vi "Find Object Layout Index by UID.vi"(8 "error in (no error)":errorcluster, 9 "unique name":i32, 10 "object ID list in":variant, 11 "object layouts in":refnum<class "Object Layout.lvclass">[](array[class])) -> (0 "error out":errorcluster, 1 "found?":bool, 2 "object ID list out":variant, 3 "object layouts out":refnum<class "Object Layout.lvclass">[](array[class]), 5 "object layout index":i32)   [LabVIEW 2010, in "NI_SE_Front Panel Layout.lvlib"]
uses:
  NI_SE_Front Panel Layout.lvlib
  Object Layout Classes/Object Layout/Object Layout.lvclass
  Object Layout Classes/Object Layout/Object Layout.lvclass/Object Layout.ctl
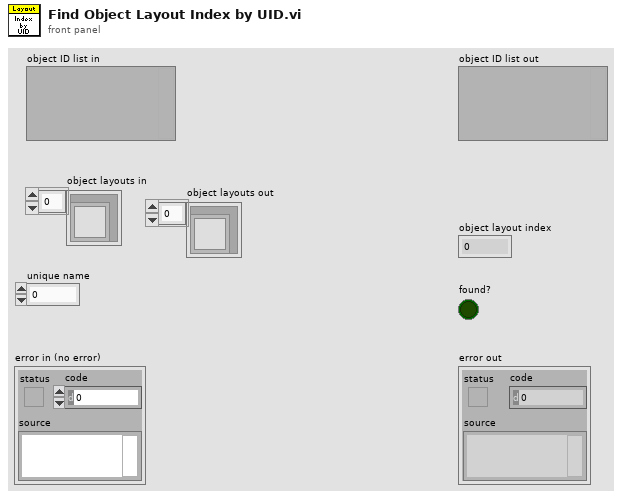
[diagram p1: front panel]
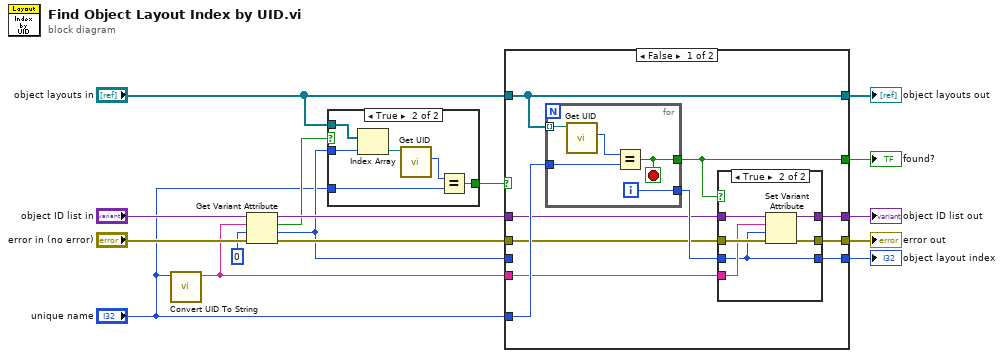
[diagram p0: block diagram]
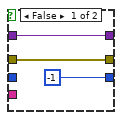
[diagram p3: hidden frame]
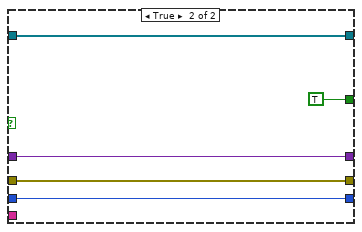
[diagram p4: hidden frame]
diagram:
  n1 = call "Convert UID To String.vi"("UID"="unique name") -> ("UID string"=w2:string)  [unwired: 10 in]
  n2 = Get Variant Attribute(Variant="object ID list in", name=w2, default value (empty Variant)=0, error in="error in (no error)") -> (duplicate Variant=w8:variant, found=w5:bool, value=w6:i32, error out=w7:errorcluster)
  n3 = case shown="True" w5 {
    tunnel: "object layouts in" -> [_ w22]
    tunnel: w6 -> [_ w21]
    tunnel: "unique name" -> [_ w20]
    tunnel: [_ w19] -> w4
    frame False {
    }
    frame True {
      n4 = Index Array(array=w22, index=w21) -> (element=w18:refnum<class "Object Layout.lvclass">)
      n5 = call "Get UID.vi"("Object Layout in"=w18) -> ("UID"=w17:i32)  [unwired: 8 in, 2 out]
      n6 = Equal?(x=w17, y=w20) -> (x = y?=w19:bool)
    }
  }
  n7 = case shown="False" w4 {
    tunnel: "object layouts in" -> [w23 w47]
    tunnel: w8 -> [w27 w51]
    tunnel: [w26 w51] -> w10
    tunnel: w6 -> [_ w48]
    tunnel: w7 -> [w24 w50]
    tunnel: [w30 w50] -> w13
    tunnel: [w31 w48] -> w15
    tunnel: [w25 TRUE] -> w14
    tunnel: "unique name" -> [w32 _]
    tunnel: w2 -> [w29 _]
    tunnel: [w23 w47] -> w1
    frame False {
      n8 = for {
        tunnel: w23 -> [w43] mode=indexing
        tunnel: [w46] -> w25
        tunnel: w32 -> [w45]
        tunnel: [w44] -> w28
        i -> [w44]
        stop <- w46 stop-if-true
        n9 = call "Get UID.vi"("Object Layout in"=w43) -> ("UID"=w42:i32)  [unwired: 8 in, 2 out]
        n10 = Equal?(x=w42, y=w45) -> (x = y?=w46:bool)
      }
      n11 = case shown="True" w25 {
        tunnel: [-1 w36] -> w31
        tunnel: [w34 w41] -> w30
        tunnel: w24 -> [w34 w40]
        tunnel: w27 -> [w35 w39]
        tunnel: w29 -> [_ w38]
        tunnel: w28 -> [_ w36]
        tunnel: [w35 w37] -> w26
        frame False {
        }
        frame True {
          n12 = Set Variant Attribute(Variant=w39, name=w38, value=w36, error in=w40) -> (Variant out=w37:variant, error out=w41:errorcluster)  [unwired: 1 out]
        }
      }
    }
    frame True {
    }
  }
  "error out" <- w13
  "object layout index" <- w15
  "found?" <- w14
  "object ID list out" <- w10
  "object layouts out" <- w1
